vi "MHL Queue Ref Holder.vi"(0 "Message Queue In":refnum<queue>, 3 "error in":errorcluster, 6 "Action":enum16{"GET", "SET"}(ring)) -> (7 "Input Message Queue":refnum<queue>, 10 "error out":errorcluster)   [LabVIEW 2015]
doc: "Holds UI queue reference to enqueue messages without wiring."
uses:
  Message Queue/Message Cluster.ctl
  Message Queue/Message Queue.lvlib
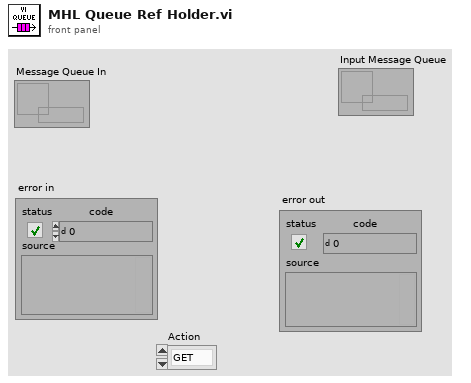
[diagram p1: front panel]
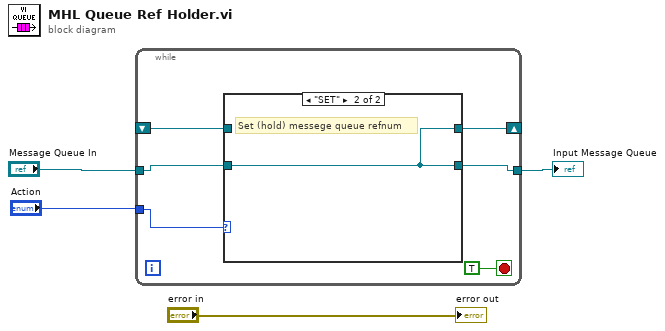
[diagram p0: block diagram]
diagram:
  n1 = while {
    tunnel: "Message Queue In" -> [w9]
    tunnel: [w6] -> w3
    tunnel: "Action" -> [w10]
    shift-right: [w8] -> _
    shift-left: _ -> [w7]
    stop <- TRUE stop-if-true
    n2 = case shown="\"SET\"" w10 {
      tunnel: w9 -> [_ w12]
      tunnel: [w11 w12] -> w6
      tunnel: [w11 w12] -> w8
      tunnel: w7 -> [w11 _]
      frame "GET", Default {
        # "Get (release) messege queue refnum"
      }
      frame "SET" {
        # "Set (hold) messege queue refnum"
      }
    }
  }
  "Input Message Queue" <- w3
  "error out" <- "error in"
